vi "decode_channel.vi"(8 "offset":u32, 9 "channel decoding":T1, 10 "port B":u8, 11 "port A":u8) -> (3 "channel value":u32)   [LabVIEW 2011]
uses:
  typedefs/channel_decoding_enum.ctl
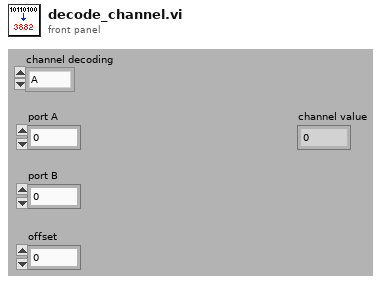
[diagram p1: front panel]
types:
  T1 = typedef "channel_decoding_enum.ctl" = enum16{"A", "B"}
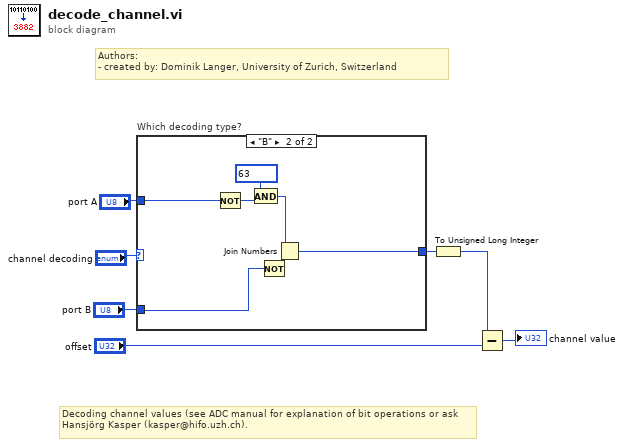
[diagram p0: block diagram]
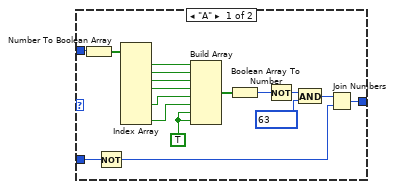
[diagram p2: hidden frame]
diagram:
  # "Authors: \n- created by: Dominik Langer, University of Zurich, Switzerland"
  # "Decoding channel values (see ADC manual for explanation of bit operations or ask Hansjörg Kasper (kasper@hifo.uzh.ch)."
  n1 = case "Which decoding type?" shown="\"B\"" "channel decoding" {
    tunnel: "port B" -> [w11 w25]
    tunnel: "port A" -> [w10 w26]
    tunnel: [w8 w29] -> w4
    frame "A" {
      w9 = TRUE
      n2 = Number To Boolean Array(number=w10) -> (Boolean array=w23:bool[])
      n3 = Not(x=w11) -> (.not. x?=w14:u8)
      n4 = Index Array(array=w23) -> (element #1=w22:bool, element #2=w21:bool, element #3=w20:bool, element #4=w19:bool, element #6=w18:bool, element #8=w17:bool)  [unwired: 8 in, 2 out]
      n5 = Build Array(w22, w21, w20, w19, w18, w17, w9, w9) -> (w16:bool[])
      n6 = Boolean Array To Number(Boolean array=w16) -> (number=w15:u8)
      n7 = Not(x=w15) -> (.not. x?=w24:u8)
      n8 = And(x=w24, y=u8 63 ("x")) -> (x .and. y?=w12:u8)
      n9 = Join Numbers(hi=w12, lo=w14) -> ((hi.lo)=w8:u16)
    }
    frame "B" {
      n10 = Not(x=w26) -> (.not. x?=w30:u8)
      n11 = And(x=u8 63, y=w30) -> (x .and. y?=w27:u8)
      n12 = Not(x=w25) -> (.not. x?=w31:u8)
      n13 = Join Numbers(hi=w27, lo=w31) -> ((hi.lo)=w29:u16)
    }
  }
  n14 = To Unsigned Long Integer(number=w4) -> (unsigned 32bit integer=w3:u32)
  n15 = Subtract(x=w3, y="offset") -> (x-y=→"channel value":u32)
